vi "Interpolation.vi"(1 "Distance Objective":dbl=60.0 format="%#_13g", 2 "Start Distance":dbl, 3 "Current Encoder Distance":dbl) -> (0 "Motor Output":dbl)   [LabVIEW 2017]
panel:
  # "Interpolation\nTeam 34 Rockets"
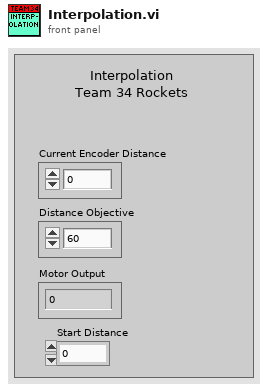
[diagram p1: front panel]
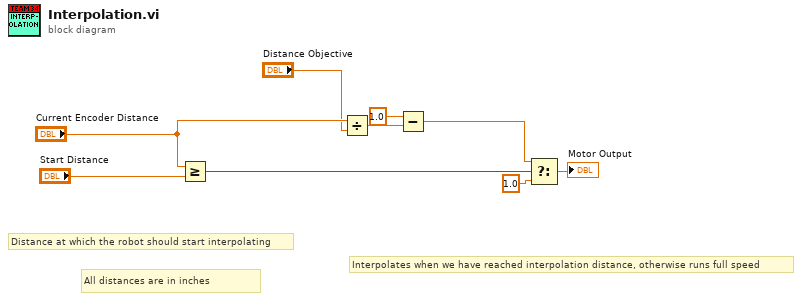
[diagram p0: block diagram]
diagram:
  # "All distances are in inches"
  # "Interpolates when we have reached interpolation distance, otherwise runs full speed"
  # "Distance at which the robot should start interpolating"
  n1 = Greater Or Equal?(x="Current Encoder Distance", y="Start Distance") -> (x >= y?=w7:bool)
  n2 = Divide(x="Current Encoder Distance", y="Distance Objective") -> (x/y=w2:dbl)
  n3 = Subtract(x=1.0, y=w2) -> (x-y=w3:dbl)
  n4 = Select(t=w3, s=w7, f=1.0) -> (s? t:f=→"Motor Output":dbl)
